vi "Write Event Name.vi"(8 "error in (no error)":errorcluster, 10 "Event Name":string, 11 "TAS_Event in":refnum<class "TAS_Event.lvclass">) -> (0 "error out":errorcluster, 3 "TAS_Event out":refnum<class "TAS_Event.lvclass">)   [LabVIEW 2012, in "TAS_Event.lvclass"]
uses:
  TAS_Event.lvclass
  TAS_Event.lvclass/TAS_Event.ctl
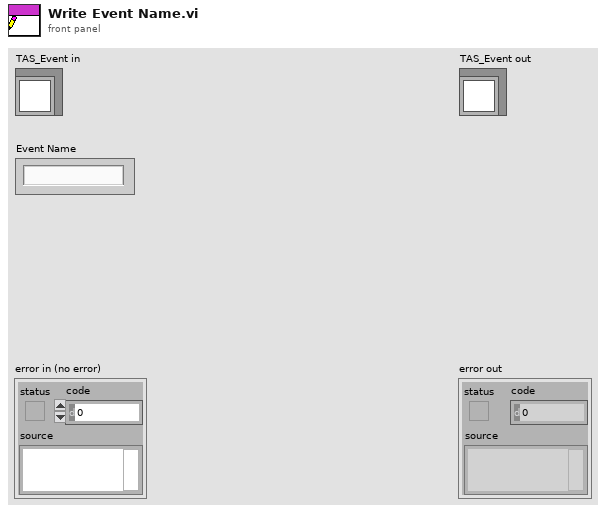
[diagram p1: front panel]
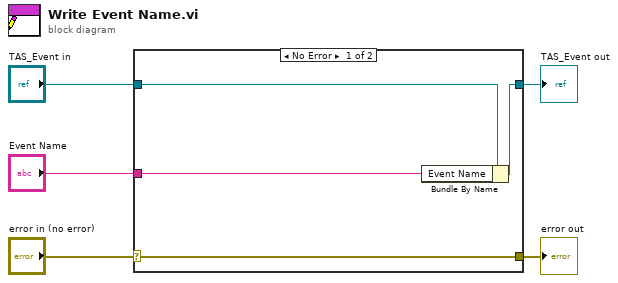
[diagram p0: block diagram]
diagram:
  n1 = case shown="No Error" "error in (no error)" {
    selector: "error in (no error)" -> [w9 w10]
    tunnel: [w9 w10] -> w4
    tunnel: [w7 w11] -> w2
    tunnel: "TAS_Event in" -> [w8 w11]
    tunnel: "Event Name" -> [w6 _]
    frame No Error {
      n2 = Bundle By Name(cluster=w8, "Event Name"=w6) -> (w7:refnum<class "TAS_Event.lvclass">)
    }
    frame Error {
    }
  }
  "error out" <- w4
  "TAS_Event out" <- w2
